vi "Turbulence_2.0.vi"() -> ()   [LabVIEW 2018]
uses:
  <instrlib>/Mercury iXX/Mercury iXX.lvlib
  <instrlib>/Quantum Composers 9000 Series 2.08/Quantum Composers 9000 Series.lvlib
  <userlib>/LightField Add-in and Automation SDK/Samples/LabVIEW Automation/lightfield-automation-labview/LightField Automation.lvclass
  <instrlib>/Mercury iXX/Public/Libraries/Temperature/Signals/Read/Temperature (Read).vi
  <instrlib>/Mercury iXX/Public/Libraries/Temperature.lvlib
  <instrlib>/Mercury iXX/Public/Libraries/Temperature/Open/Open Temperature Device.vi
  <instrlib>/Mercury iXX/Public/Libraries/System/Read/Catalogue (Read).vi
  <instrlib>/Mercury iXX/Public/Libraries/System.lvlib
  <instrlib>/Mercury iXX/Public/Libraries/System/Open/Open System.vi
  <vilib>/Utility/file.llb/Write Delimited Spreadsheet (string).vi
  <instrlib>/Mercury iXX/Public/Controls/Comms Transport Layer.ctl
  <instrlib>/Mercury iXX/Public/Controls/Unit String.ctl
panel:
  out "Array":string[](array[string])
  out "Array 2":string[](array[string])
  in  "?":bool
  in  "Turbulence Experiment":T1(tab)
  in  "VISA resource name":refnum<visa-resource-name>
  in  "Comms Layer":T2
  out "error out":errorcluster
  in  "Read Interval (s)":sgl=1.0 min=0.25 max=1000 step=0.25 format="%.2f"
  in  "Record Temperature Data":bool
  out "Unit":T3
  out "Temperature":dbl
  in  "Experiment Name":string="Experiment1"
  in  "Repetitive Gate Width (us)":dbl
  in  "Intensifier Gain":i32
  in  "Start":bool
  in  "?":bool
  in  "Time between frames":i32=500
  in  "On Chip Accumulations 2":i32=6
  in  "Number of Frames 2":i32
  in  "Data folder":path=path "C:/Data"
  in  "Oscilloscope":refnum<visa-resource-name>="USB0::0x0699::0x03A6::C016710::INSTR"
  in  "Pulse generater":refnum<visa-resource-name>="COM3"
  # "Stop Oscilloscope"
  # "Stop Lightfield"
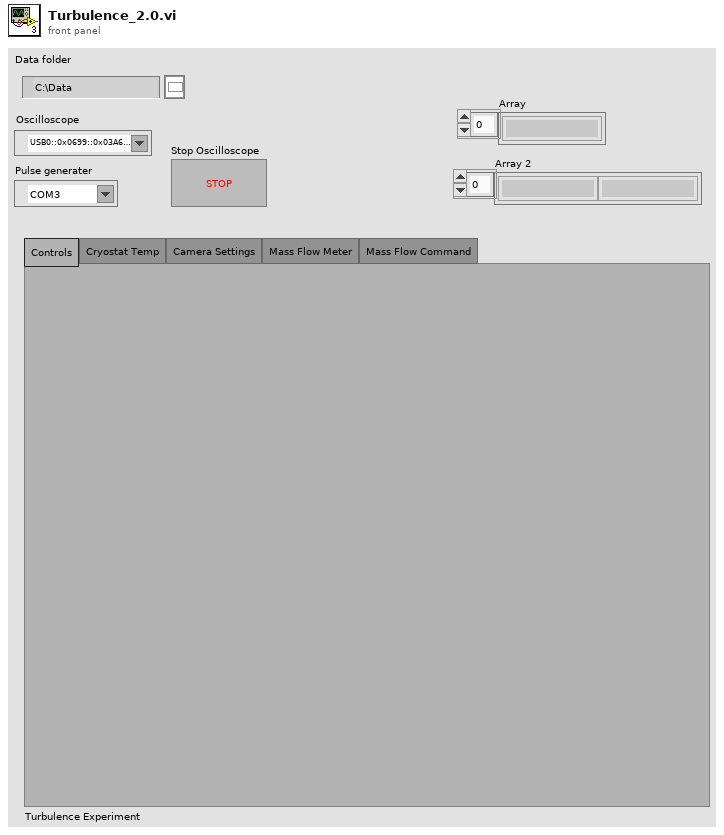
[diagram p1: front panel]
types:
  T1 = enum32{"Controls", "Cryostat Temp", "Camera Settings", "Mass Flow Meter", "Mass Flow Command"}
  T2 = typedef "Mercury iXX.lvlib/Comms Transport Layer.ctl" = enum16{"Ethernet TCP/IP", "USB", "ISOBus - RS-232", "GPIB"}
  T3 = typedef "Mercury iXX.lvlib/Unit String.ctl" = string
  T4 = typedef "Mercury iXX.lvlib/Mercury Reference.ctl" = cluster{"Comms":refnum<visa-resource-name>, "Device ID":string[], "Comms Layer":T2, "Command":string, "Query reference":T5}
  T5 = typedef "Mercury iXX.lvlib/Query Dynamic Reference.ctl" = refnum<vi>
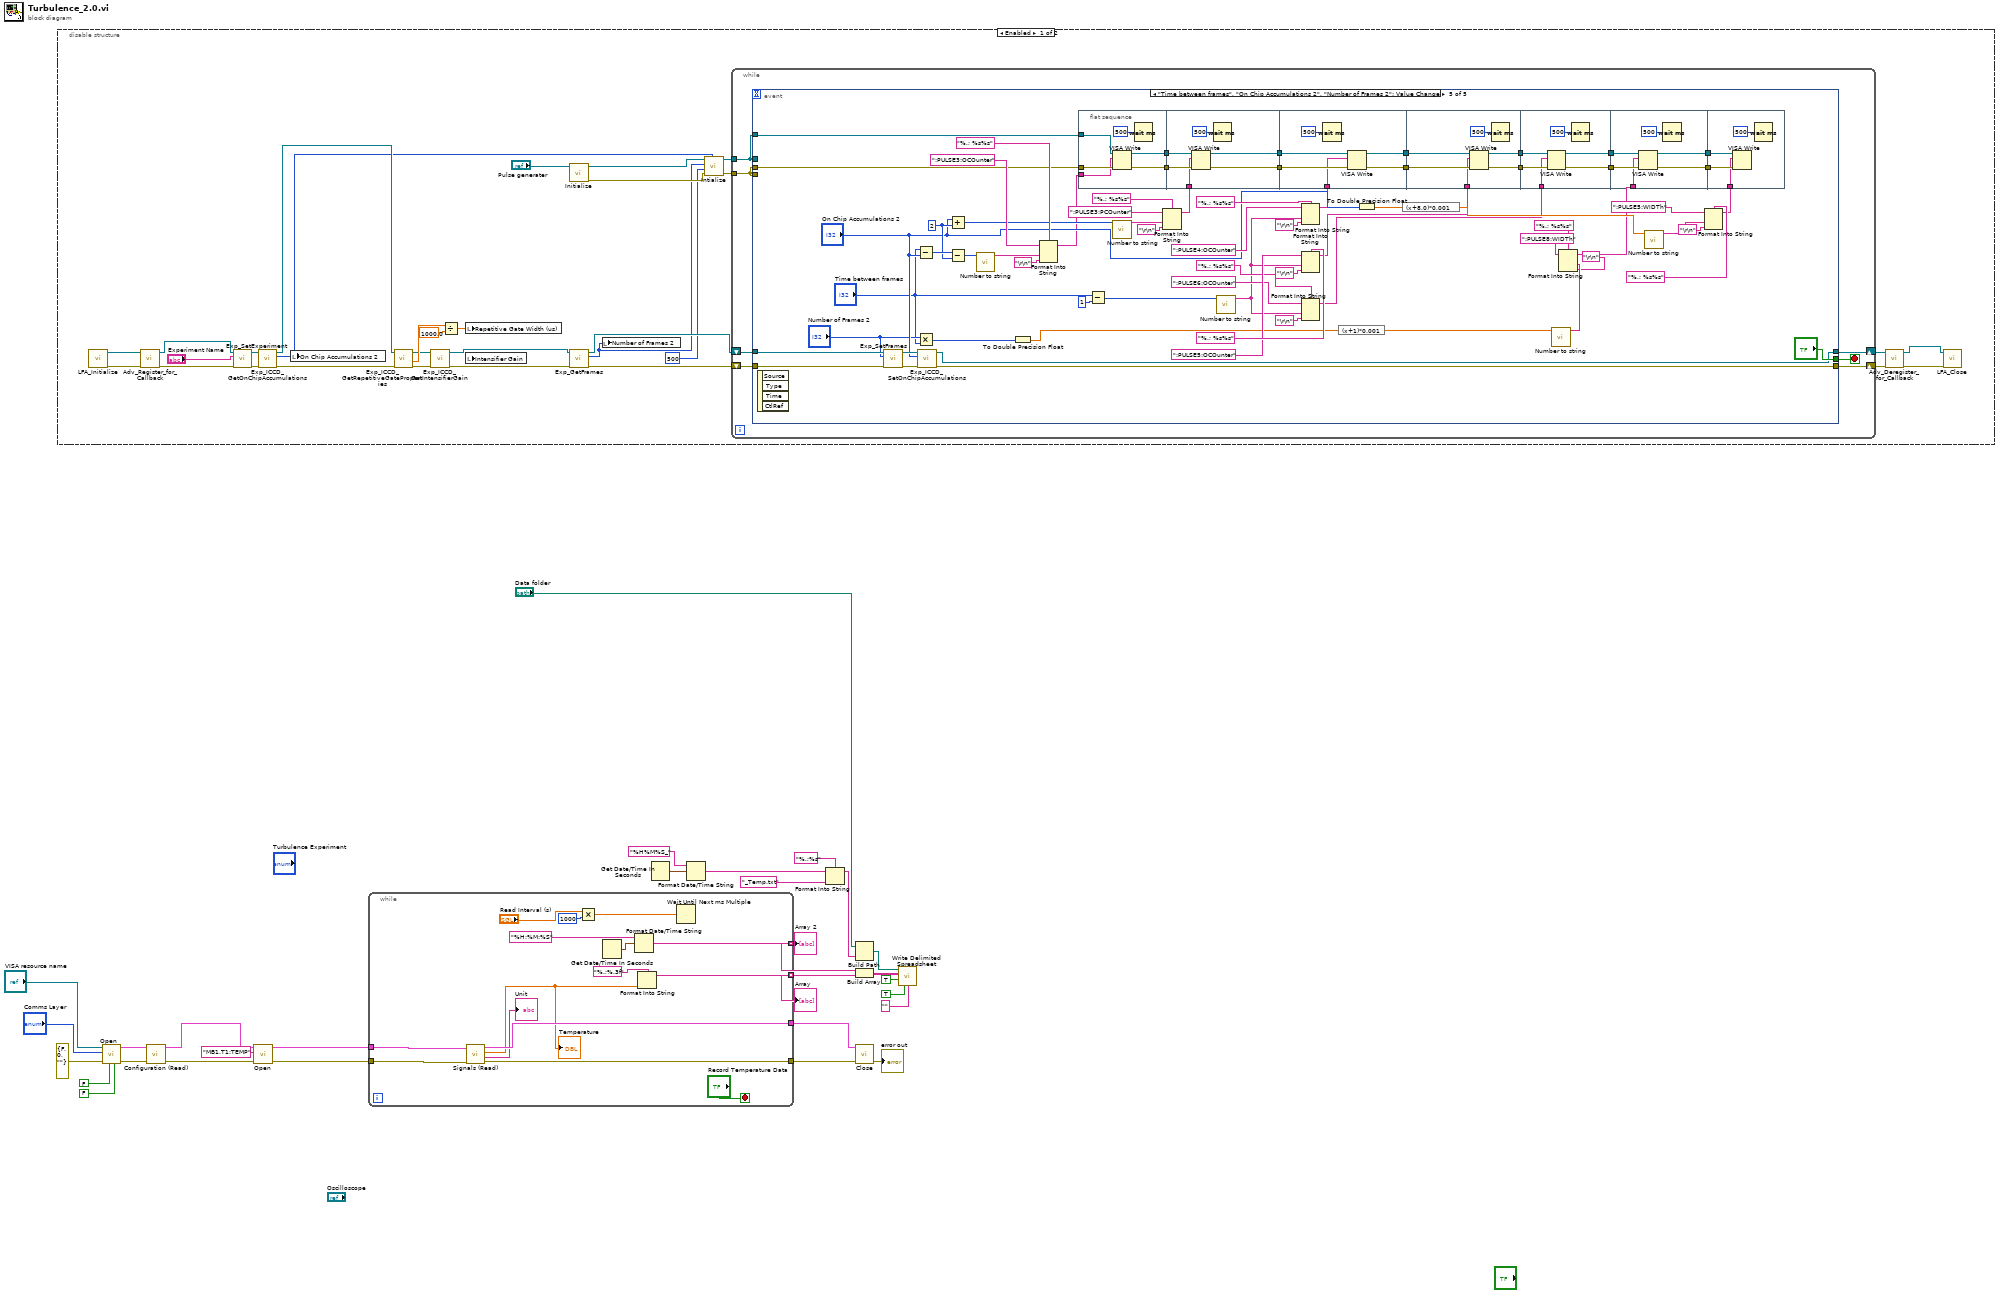
[diagram p0: block diagram]
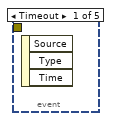
[diagram p2: hidden frame]
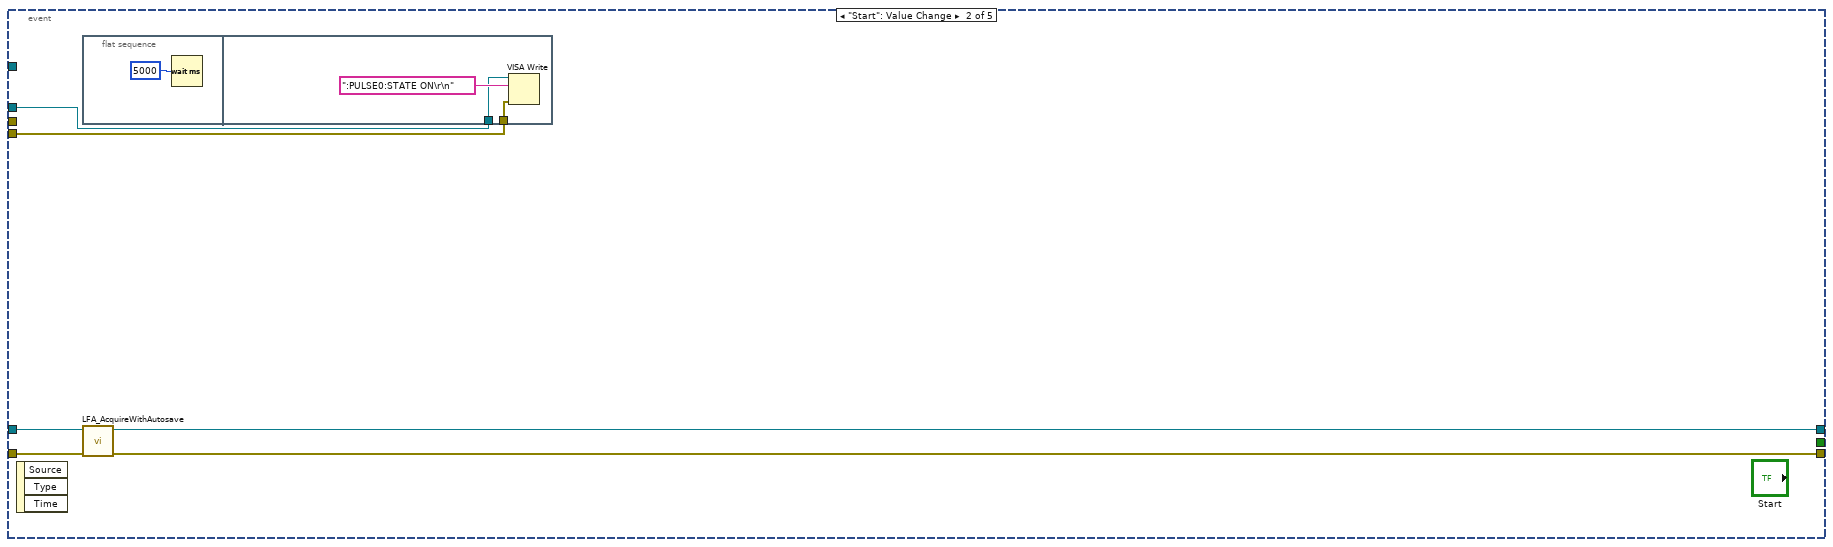
[diagram p3: hidden frame]
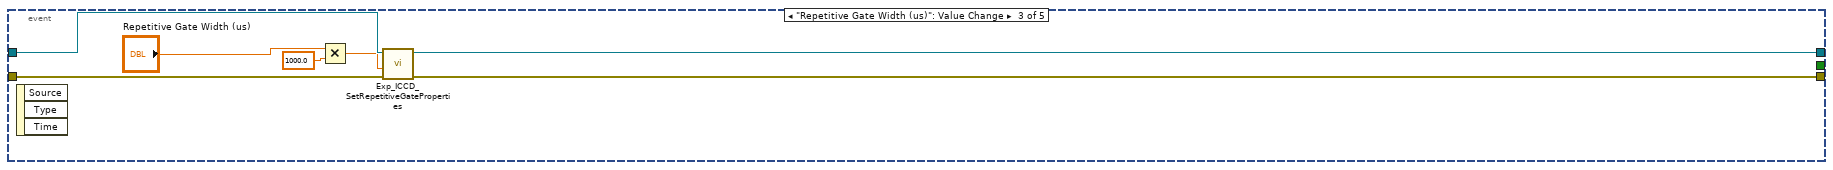
[diagram p4: hidden frame]
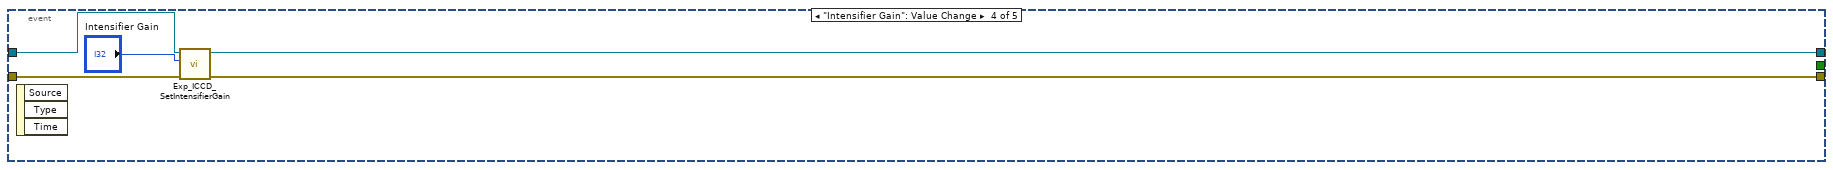
[diagram p5: hidden frame]
diagram:
  n1 = disable-structure shown="Enabled" {
    frame Enabled {
      n2 = call <userlib>:"LFA_Initialize.vi"() -> ("error out"=w30:errorcluster, "LightField Automation out"=w31:refnum<class "LightField Automation.lvclass">)  [unwired: 10 in]
      n3 = call <userlib>:"Adv_Register_for_Callback.vi"("error in (no error)"=w30, "LightField Automation in"=w31) -> ("error out"=w55:errorcluster, "LightField Automation out"=w56:refnum<class "LightField Automation.lvclass">)  [unwired: 8 in]
      n4 = call <userlib>:"Exp_SetExperiment.vi"("error in (no error)"=w55, "ExperimentName"="Experiment Name", "LightField Automation in"=w56) -> ("error out"=w51:errorcluster, "LightField Automation out"=w52:refnum<class "LightField Automation.lvclass">)  [unwired: 7 in]
      n5 = call <userlib>:"Exp_ICCD_GetOnChipAccumulations.vi"("error in (no error)"=w51, "LightField Automation in"=w52) -> ("error out"=w49:errorcluster, "On Chip Accumulations"=w34:i32, "LightField Automation out"=w50:refnum<class "LightField Automation.lvclass">)  [unwired: 7 in]
      n6 = local write "On Chip Accumulations 2"(w34) -> ()
      n7 = call <userlib>:"Exp_ICCD_GetRepetitiveGateProperties.vi"("error in (no error)"=w49, "LightField Automation in"=w50) -> ("error out"=w44:errorcluster, "Repetitive Gate Width (ns)"=w48:dbl, "LightField Automation out"=w45:refnum<class "LightField Automation.lvclass">)  [unwired: 6 in, 1 out]
      n8 = call <userlib>:"Exp_ICCD_GetIntensifierGain.vi"("error in (no error)"=w44, "LightField Automation in"=w45) -> ("error out"=w42:errorcluster, "LightField Automation out"=w43:refnum<class "LightField Automation.lvclass">)  [unwired: 7 in, 1 out]
      n9 = Divide(x=w48, y=1000.0) -> (x/y=w46:dbl)
      n10 = local write "Repetitive Gate Width (us)"(w46) -> ()
      n11 = local read "Intensifier Gain"() -> ()  [unwired: 1 in]
      n12 = call <instrlib>:"Initialize.vi"("VISA resource name"="Pulse generater") -> ("error out"=w38:errorcluster, "VISA resource name out"=w39:refnum<visa-resource-name>)  [unwired: 9 in]
      n13 = call <userlib>:"Exp_GetFrames.vi"("error in (no error)"=w42, "LightField Automation in"=w43) -> ("error out"=w41:errorcluster, "Frames"=w35:i32, "LightField Automation out"=w40:refnum<class "LightField Automation.lvclass">)  [unwired: 7 in]
      n14 = local write "Number of Frames 2"(w35) -> ()
      n15 = call "Intialize.vi"("On Chip Accumulations 3"=w34, "error in (no error)"=w38, "Time between frames 2"=500, "Number of Frames 3"=w35, "VISA resource name"=w39) -> ("error out"=w36:errorcluster, "VISA resource name out"=w37:refnum<visa-resource-name>)  [unwired: 5 in]
      n16 = while {
        tunnel: w37 -> [w60]
        tunnel: w36 -> [w61]
        shift-right: [w65] -> w54
        shift-left: w40 -> [w63]
        shift-right: [w66] -> w53
        shift-left: w41 -> [w64]
        stop <- w62 stop-if-true
        n17 = event shown="[4] \"Time between frames\", \"On Chip Accumulations 2\", \"Number of Frames 2\": Value Change" {
          selector: _ -> [_ _ _ _ _]
          dyn-events: _ -> [_ _ _ _ _]
          timeout: _ -> [_ _ _ _ _]
          tunnel: w61 -> [_ w72 _ _ _]
          tunnel: w60 -> [_ w69 _ _ _]
          tunnel: w64 -> [_ w71 w82 w86 w124]
          tunnel: w63 -> [_ w70 w83 w87 w125]
          tunnel: [_ w67 w80 w84 w120] -> w66
          tunnel: [_ w68 w81 w85 w121] -> w65
          tunnel: [_ _ _ _ "?"] -> w62
          tunnel: w61 -> [_ _ _ _ w109]
          tunnel: w60 -> [_ _ _ _ w107]
          event Timeout {
            n18 = event-data() -> ()  [unwired: 1 in, 3 out]
          }
          event "Start": Value Change {
            n19 = event-data() -> ()  [unwired: 1 in, 3 out]
            n20 = flat-sequence {
              tunnel: w72 -> [w76]
              tunnel: w69 -> [w74]
              frame #0 {
                n21 = Wait (ms)(milliseconds to wait=5000) -> ()  [unwired: 1 out]
              }
              frame #1 {
                n22 = VISA Write(VISA resource name=w74, write buffer=":PULSE0:STATE ON\r\n" ("format string"), error in (no error)=w76) -> ()  [unwired: 3 out]
              }
            }
            n23 = call <userlib>:"LFA_AcquireWithAutosave.vi"("error in (no error)"=w71, "LightField Automation in"=w70) -> ("error out"=w67:errorcluster, "LightField Automation out"=w68:refnum<class "LightField Automation.lvclass">)  [unwired: 7 in, 1 out]
          }
          event "Repetitive Gate Width (us)": Value Change {
            n24 = event-data() -> ()  [unwired: 1 in, 3 out]
            n25 = Multiply(x="Repetitive Gate Width (us)", y=1000.0) -> (x*y=w77:dbl)
            n26 = call <userlib>:"Exp_ICCD_SetRepetitiveGateProperties.vi"("error in (no error)"=w82, "Repetitive Gate Width (ns)"=w77, "LightField Automation in"=w83) -> ("error out"=w80:errorcluster, "LightField Automation out"=w81:refnum<class "LightField Automation.lvclass">)  [unwired: 7 in]
          }
          event "Intensifier Gain": Value Change {
            n27 = event-data() -> ()  [unwired: 1 in, 3 out]
            n28 = call <userlib>:"Exp_ICCD_SetIntensifierGain.vi"("error in (no error)"=w86, "Intensifier Gain"="Intensifier Gain", "LightField Automation in"=w87) -> ("error out"=w84:errorcluster, "LightField Automation out"=w85:refnum<class "LightField Automation.lvclass">)  [unwired: 7 in]
          }
          event "Time between frames", "On Chip Accumulations 2", "Number of Frames 2": Value Change {
            w149 = 2 ("y")
            n29 = event-data() -> ()  [unwired: 1 in, 4 out]
            n30 = call <userlib>:"Exp_SetFrames.vi"("error in (no error)"=w124, "Number of Frames"="Number of Frames 2", "LightField Automation in"=w125) -> ("error out"=w122:errorcluster, "LightField Automation out"=w123:refnum<class "LightField Automation.lvclass">)  [unwired: 7 in]
            n31 = Subtract(x="Time between frames", y="On Chip Accumulations 2") -> (x-y=w151:i32)
            n32 = Multiply(x="Number of Frames 2", y="Time between frames") -> (x*y=w110:i32)
            n33 = call <userlib>:"Exp_ICCD_SetOnChipAccumulations.vi"("error in (no error)"=w122, "On Chip Accumulations"="On Chip Accumulations 2", "LightField Automation in"=w123) -> ("error out"=w120:errorcluster, "LightField Automation out"=w121:refnum<class "LightField Automation.lvclass">)  [unwired: 7 in]
            n34 = Add(x="On Chip Accumulations 2", y=w149) -> (x+y=w145:i32)
            n35 = Subtract(x=w151, y=w149) -> (x-y=w150:i32)
            n36 = call "Number to string.vi"("Numeric"=w150) -> ("Shortest String"=w155:string)  [unwired: 10 in]
            n37 = To Double Precision Float(number=w110) -> (double precision float=w131:dbl)
            n38 = Format Into String(format string="%.; %s%s", initial string=":PULSE3:OCOunter" ("format string"), w155, "\r\n" ("format string")) -> (resulting string=w108:string)  [unwired: 1 in, 1 out]
            n39 = flat-sequence {
              tunnel: w109 -> [w162]
              tunnel: w108 -> [w161]
              tunnel: w107 -> [w160]
              tunnel: [w159] -> w106
              tunnel: [w158] -> w104
              tunnel: w106 -> [w167]
              tunnel: w105 -> [w166]
              tunnel: w104 -> [w165]
              tunnel: [w164] -> w103
              tunnel: [w163] -> w101
              tunnel: w103 -> [w174]
              tunnel: w102 -> [w173]
              tunnel: w101 -> [w172]
              tunnel: [w171] -> w100
              tunnel: [w170] -> w98
              tunnel: w100 -> [w180]
              tunnel: w99 -> [w179]
              tunnel: w98 -> [w178]
              tunnel: [w177] -> w97
              tunnel: [w176] -> w95
              tunnel: w97 -> [w186]
              tunnel: w96 -> [w185]
              tunnel: w95 -> [w184]
              tunnel: [w183] -> w94
              tunnel: [w182] -> w92
              tunnel: w94 -> [w192]
              tunnel: w93 -> [w191]
              tunnel: w92 -> [w190]
              tunnel: [w189] -> w91
              tunnel: [w188] -> w89
              tunnel: w91 -> [w196]
              tunnel: w90 -> [w195]
              tunnel: w89 -> [w194]
              frame #0 {
                n40 = VISA Write(VISA resource name=w160, write buffer=w161, error in (no error)=w162) -> (VISA resource name out=w158:refnum<visa-resource-name>, error out=w159:errorcluster)  [unwired: 1 out]
                n41 = Wait (ms)(milliseconds to wait=500) -> ()  [unwired: 1 out]
              }
              frame #1 {
                n42 = VISA Write(VISA resource name=w165, write buffer=w166, error in (no error)=w167) -> (VISA resource name out=w163:refnum<visa-resource-name>, error out=w164:errorcluster)  [unwired: 1 out]
                n43 = Wait (ms)(milliseconds to wait=500) -> ()  [unwired: 1 out]
              }
              frame #2 {
                n44 = Wait (ms)(milliseconds to wait=500) -> ()  [unwired: 1 out]
                n45 = VISA Write(VISA resource name=w172, write buffer=w173, error in (no error)=w174) -> (VISA resource name out=w170:refnum<visa-resource-name>, error out=w171:errorcluster)  [unwired: 1 out]
              }
              frame #3 {
                n46 = VISA Write(VISA resource name=w178, write buffer=w179, error in (no error)=w180) -> (VISA resource name out=w176:refnum<visa-resource-name>, error out=w177:errorcluster)  [unwired: 1 out]
                n47 = Wait (ms)(milliseconds to wait=500) -> ()  [unwired: 1 out]
              }
              frame #4 {
                n48 = VISA Write(VISA resource name=w184, write buffer=w185, error in (no error)=w186) -> (VISA resource name out=w182:refnum<visa-resource-name>, error out=w183:errorcluster)  [unwired: 1 out]
                n49 = Wait (ms)(milliseconds to wait=500) -> ()  [unwired: 1 out]
              }
              frame #5 {
                n50 = VISA Write(VISA resource name=w190, write buffer=w191, error in (no error)=w192) -> (VISA resource name out=w188:refnum<visa-resource-name>, error out=w189:errorcluster)  [unwired: 1 out]
                n51 = Wait (ms)(milliseconds to wait=500) -> ()  [unwired: 1 out]
              }
              frame #6 {
                n52 = VISA Write(VISA resource name=w194, write buffer=w195, error in (no error)=w196) -> ()  [unwired: 3 out]
                n53 = Wait (ms)(milliseconds to wait=500) -> ()  [unwired: 1 out]
              }
            }
            n54 = Subtract(x="Time between frames", y=1) -> (x-y=w142:i32)
            n55 = call "Number to string.vi"("Numeric"=w145) -> ("Shortest String"=w148:string)  [unwired: 10 in]
            n56 = Format Into String(format string="%.; %s%s", initial string=":PULSE3:PCOunter" ("format string"), w148, "\r\n" ("format string")) -> (resulting string=w105:string)  [unwired: 1 in, 1 out]
            n57 = call "Number to string.vi"("Numeric"=w142) -> ("Shortest String"=w132:string)  [unwired: 10 in]
            n58 = Format Into String(format string="%.; %s%s", initial string=":PULSE4:OCOunter" ("format string"), w132, "\r\n" ("format string")) -> (resulting string=w102:string)  [unwired: 1 in, 1 out]
            n59 = Format Into String(format string="%.; %s%s", initial string=":PULSE5:OCOunter" ("format string"), w132, "\r\n" ("format string")) -> (resulting string=w99:string)  [unwired: 1 in, 1 out]
            n60 = Format Into String(format string="%.; %s%s", initial string=":PULSE6:OCOunter" ("format string"), w132, "\r\n" ("format string")) -> (resulting string=w96:string)  [unwired: 1 in, 1 out]
            n61 = expression code="(x+1)*0.001"(w131) -> (w128:dbl)
            n62 = To Double Precision Float(number="On Chip Accumulations 2") -> (double precision float=w118:dbl)
            n63 = expression code="(x+8.0)*0.001"(w118) -> (w113:dbl)
            n64 = call "Number to string.vi"("Numeric"=w128) -> ("Shortest String"=w127:string)  [unwired: 10 in]
            n65 = Format Into String(format string="%.; %s%s", initial string=":PULSE8:WIDTh" ("format string"), w127, "\r\n" ("format string")) -> (resulting string=w93:string)  [unwired: 1 in, 1 out]
            n66 = call "Number to string.vi"("Numeric"=w113) -> ("Shortest String"=w115:string)  [unwired: 10 in]
            n67 = Format Into String(format string="%.; %s%s", initial string=":PULSE5:WIDTh" ("format string"), w115, "\r\n" ("format string")) -> (resulting string=w90:string)  [unwired: 1 in, 1 out]
          }
        }
      }
      n68 = call <userlib>:"Adv_Deregister_for_Callback.vi"("error in (no error)"=w53, "LightField Automation in"=w54) -> ("error out"=w32:errorcluster, "LightField Automation out"=w58:refnum<class "LightField Automation.lvclass">)  [unwired: 8 in]
      n69 = call <userlib>:"LFA_Close.vi"("error in (no error)"=w32, "LightField Automation in"=w58) -> ()  [unwired: 8 in, 2 out]
    }
    frame Disabled {
    }
  }
  n70 = call-poly <instrlib>:"Open.vi"("Clear Previous Connections (False)"=FALSE, "ID Query (True)"=FALSE, "error in (no error)"=errorcluster {"status"=FALSE, "code"=0, "source"=""}, "Comms Layer"="Comms Layer", "VISA resource name"="VISA resource name") -> ("error out"=w25:errorcluster, "Mercury Reference Out"=w26:T4)  [unwired: 2 in, 3 out]
  n71 = call-poly <instrlib>:"Configuration (Read).vi"("error in"=w25, "Mercury Reference In"=w26) -> ("error out"=w23:errorcluster, "Mercury Reference Out"=w24:T4)  [unwired: 6 in, 2 out]
  n72 = call-poly <instrlib>:"Open.vi"("error in (no error)"=w23, "Device Identifier"="MB1.T1:TEMP", "Mercury Reference In"=w24) -> ("error out"=w2:errorcluster, "Mercury Reference Out"=w1:T4)  [unwired: 7 in]
  n73 = while {
    tunnel: [w211] -> w22
    tunnel: [w210] -> w21
    tunnel: [w199] -> w15 mode=indexing
    tunnel: [w202] -> w16 mode=indexing
    tunnel: w2 -> [w198]
    tunnel: w1 -> [w197]
    stop <- "Record Temperature Data" stop-if-true
    n74 = call-poly <instrlib>:"Signals (Read).vi"("error in"=w198, "Mercury Reference In"=w197) -> ("error out"=w211:errorcluster, "Unit"=→"Unit":T3, "Temperature"=w200:dbl, "Mercury Reference Out"=w210:T4)  [unwired: 5 in, 1 out]
    "Temperature" <- w200
    n75 = Multiply(x="Read Interval (s)", y=u32 1000 ("millisecond multiple")) -> (x*y=w205:sgl)
    n76 = Get Date/Time In Seconds() -> (seconds since 1Jan1904=w203:timestamp)
    n77 = Format Date/Time String(time format string (%c)="%H:%M:%S", seconds (now)=w203) -> (date/time string=w202:string)  [unwired: 1 in]
    n78 = Format Into String(format string="%.;%.3f", w200) -> (resulting string=w199:string)  [unwired: 2 in, 1 out]
    n79 = Wait Until Next ms Multiple(millisecond multiple=w205) -> ()  [unwired: 1 out]
  }
  "Array 2" <- w16
  "Array" <- w15
  n80 = Get Date/Time In Seconds() -> (seconds since 1Jan1904=w13:timestamp)
  n81 = Format Date/Time String(time format string (%c)="%H%M%S_", seconds (now)=w13) -> (date/time string=w9:string)  [unwired: 1 in]
  n82 = Format Into String(format string="%.;%s", initial string=w9, "_Temp.txt" ("input 2")) -> (resulting string=w10:string)  [unwired: 1 in, 1 out]
  n83 = Build Path(base path="Data folder", name or relative path=w10) -> (appended path=w5:path)
  n84 = Build Array(w16, w15) -> (w4:string[][])
  n85 = call <instrlib>:"Close.vi"("error in (no error)"=w22, "Mercury Reference"=w21) -> ("error out"=→"error out":errorcluster)  [unwired: 9 in]
  n86 = call-poly <vilib>:"Write Delimited Spreadsheet.vi"("file path (dialog if empty)"=w5, "2D data"=w4, "append to file? (new file:F)"=TRUE, "transpose? (no:F)"=TRUE, "delimiter (\\t)"="" ("delimiter (\\t)")) -> ()  [unwired: 9 in, 2 out]
